vi "UTIL Update Moving Average Temp.vi"(8 "Error In":errorcluster, 10 "Data Point":dbl, 11 "Average Queue":refnum<queue>) -> (0 "Error Out":errorcluster, 3 "Moving Average":dbl)   [LabVIEW 2010]
doc: "This computes a backward Moving Average, using a fixed-length Queue to hold the last N points. The algorithm is simple -- do a Lossy Enqueue, which bumps out the oldest point, use the Get Queue Status to get the Queue contents (without emptying the Queue) and return the Mean.\n\nInput:\n Average Qyeye Fixed-length Queue of Dbl\n DataPoint Dbl\n Error In\nOutput:\n Moving Average Dbl\n Error Out"
uses:
  <vilib>/Analysis/NI_AALBase.lvlib
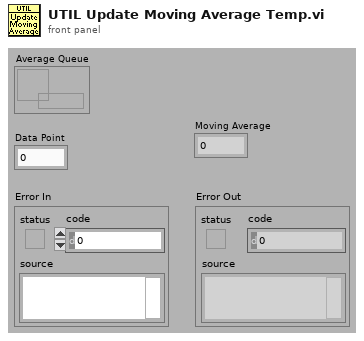
[diagram p1: front panel]
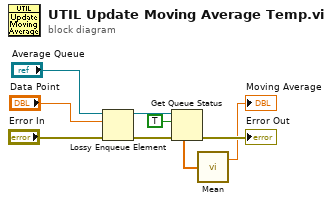
[diagram p0: block diagram]
diagram:
  n1 = Lossy Enqueue Element(queue="Average Queue", element="Data Point", error in (no error)="Error In") -> (queue out=w4:refnum<queue>, error out=w8:errorcluster)  [unwired: 2 out]
  n2 = Get Queue Status(queue=w4, return elements? (F)=TRUE, error in (no error)=w8) -> (error out=→"Error Out":errorcluster, elements=w2:dbl[])  [unwired: 6 out]
  n3 = call <vilib>:"Mean.vi"("X"=w2) -> ("mean"=→"Moving Average":dbl)  [unwired: 1 out]
